vi "Unpack JSON Message.vi"(8 "error in (no error)":errorcluster, 10 "Payload":T1) -> (0 "error out":errorcluster, 1 "Data JSON":string, 2 "ID":string)   [LabVIEW 2020, in "HTTP Server.lvlib" / "Basic WebSocket Manager.lvclass"]
uses:
  Basic WebSocket Manager.lvclass
  Basic WebSocket Manager.lvclass/Basic WebSocket Manager.ctl
  <vilib>/JDP Science/JSONtext/JSONtext.lvlib
  451c1117-54de-4ee5-b0dc-854834b80b26.vi
  WebSocket Format.ctl
  HTTP Server.lvlib
  WS Payload.ctl
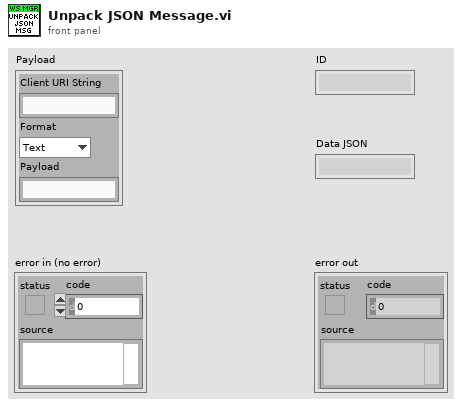
[diagram p1: front panel]
types:
  T1 = typedef "HTTP Server.lvlib/Basic WebSocket Manager.lvclass/WS Payload.ctl" = cluster{"Client URI String":string, "Format":T2, "Payload":string}
  T2 = typedef "HTTP Server.lvlib/WebSocket Format.ctl" = enum16{"Text", "Binary"}
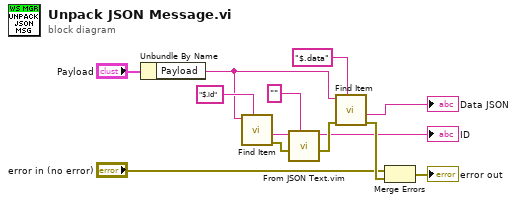
[diagram p0: block diagram]
diagram:
  n1 = Unbundle By Name("Payload") -> ("Payload"=w1:string)
  n2 = call <vilib>:"Find Item.vi"("$Path or Item Name"="$.id", "JSON"=w1) -> ("error out"=w3:errorcluster, "<JSON>"=w9:string)  [unwired: 6 in, 2 out]
  n3 = call "From JSON Text.vim"("Data Type and Default Value"="", "error in (no error)"=w3, "JSON"=w9) -> ("error out"=w12:errorcluster, "Data out"=→"ID":string)  [unwired: 7 in]
  n4 = call <vilib>:"Find Item.vi"("$Path or Item Name"="$.data", "error in (no error)"=w12, "JSON"=w1) -> ("error out"=w13:errorcluster, "<JSON>"=→"Data JSON":string)  [unwired: 5 in, 2 out]
  n5 = Merge Errors("error in (no error)", w13) -> (→"error out":errorcluster)
